vi "ReversedEngineering FindAttributeToCopy.vi"(0 "OrgClusterMembers":T2(array[cluster]), 1 "Cluster":T3, 8 "AlreadyUSedControls":i32[](array[numeric])) -> (14 "index of element":i32)   [LabVIEW 2014]
uses:
  <resource>/Framework/Providers/Open_GDS/ClassProviders/Common/CommonVIs/CommonVIs_AttributeDataType.ctl
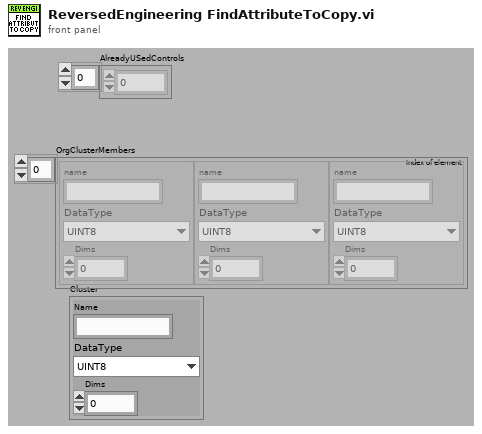
[diagram p1: front panel]
types:
  T1 = typedef "CommonVIs_AttributeDataType.ctl" = enum16{"UINT8", "INT8", "UINT16", "INT16", "UINT32", "INT32", "UINT64", "INT64", "SGL", "DBL", "EXT", "CSG", "CDB", "CXT", "TimeStamp", "STRING", "PATH", "BOOL", "ENUM", "RefNum", "VIRefNum", "LabVIEW Class", "Cluster", "Variant", "TypeDef", "Waveform", "LabVIEW Object", "Other", "void"}
  T2 = cluster{"name":string, "DataType":T1, "Dims":i32}[]
  T3 = cluster{"Name":string, "DataType":T1, "Dims":i32}
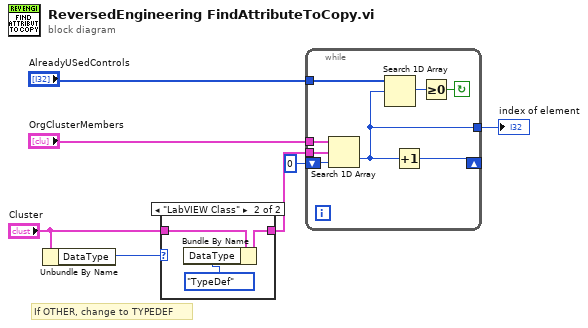
[diagram p0: block diagram]
diagram:
  # "If OTHER, change to TYPEDEF"
  n1 = Unbundle By Name("Cluster") -> ("DataType"=w1:T1)
  n2 = case shown="\"LabVIEW Class\"" w1 {
    tunnel: "Cluster" -> [w8 w11]
    tunnel: [w8 w10] -> w2
    frame Default {
    }
    frame "LabVIEW Class" {
      n3 = Bundle By Name(cluster=w11, "DataType"=CommonVIs_AttributeDataType."TypeDef" ("AttributeDataType")) -> (w10:T3)
    }
  }
  n4 = while {
    tunnel: w2 -> [w19]
    tunnel: "OrgClusterMembers" -> [w18]
    tunnel: "AlreadyUSedControls" -> [w17]
    shift-right: [w12] -> _
    shift-left: 0 -> [w14]
    tunnel: [w13] -> w5
    stop <- w15 continue-if-true
    n5 = Search 1D Array(1D array=w18, element=w19, start index (0)=w14) -> (index of element=w13:i32)
    n6 = Search 1D Array(1D array=w17, element=w13) -> (index of element=w16:i32)  [unwired: 1 out]
    n7 = Increment(x=w13) -> (x+1=w12:i32)
    n8 = Greater Or Equal To 0?(x=w16) -> (x >= 0?=w15:bool)
  }
  "index of element" <- w5
